vi "sub_ntrip_mount-point-names.vi"(11 "ntrip str":string) -> (3 "mount points":string[](array[string]))   [LabVIEW 2019]
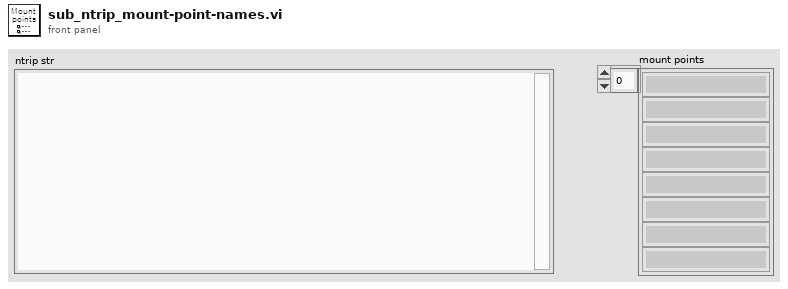
[diagram p1: front panel]
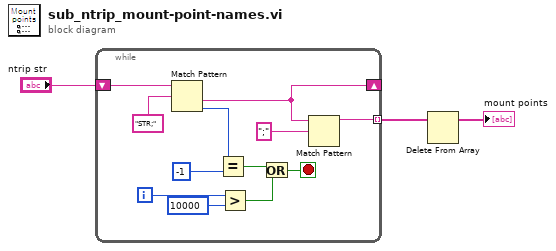
[diagram p0: block diagram]
diagram:
  n1 = while {
    shift-right: [w13] -> _
    shift-left: "ntrip str" -> [w15]
    tunnel: [w12] -> w2 mode=indexing
    i -> [w8]
    stop <- w5 stop-if-true
    n2 = Match Pattern(string=w15, regular expression="STR;" ("정규식")) -> (after substring=w13:string, offset past match=w11:i32)  [unwired: 1 in, 2 out]
    n3 = Equal?(x=w11, y=-1) -> (x = y?=w6:bool)
    n4 = Greater?(x=w8, y=10000) -> (0:w4:bool)
    n5 = Or(x=w6, y=w4) -> (x .or. y?=w5:bool)
    n6 = Match Pattern(string=w13, regular expression=";" ("정규식")) -> (before substring=w12:string)  [unwired: 1 in, 3 out]
  }
  n7 = Delete From Array(array=w2) -> (array with subset deleted=→"mount points":string[])  [unwired: 2 in, 1 out]
